vi "ArmMotorControl.vi"(8 "error in":errorcluster) -> ()   [LabVIEW 2014]
uses:
  Gantry/GantryGlobals.vi
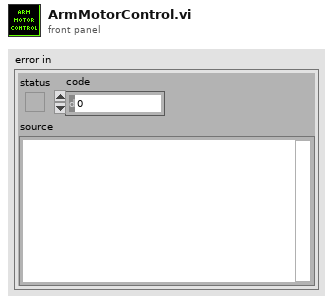
[diagram p1: front panel]
types:
  T1 = typedef "WPI_MotorControlDeviceRef.ctl" = cluster{"DeviceStatus":errorcluster, "Type":T2, "PWM":cluster{"Controller":T3, "PWM Channel":T4, "DeadBand":T5}, "CAN":cluster{"Device Number":u8, "Control Mode":T6, "Semaphore":T7, "Max Vout":dbl, "TalonSRX Control Mode":T8}, "Invert":bool, "TransformRef":T9, "InvTransformRef":T9}
  T2 = typedef "WPI_MotorControlType.ctl" = enum16{"PWM", "CAN", "CANTalonSRX"}
  T3 = typedef "FPGA_TypedefDigitalModule.ctl" = enum16{"Controller 1"}
  T4 = typedef "FPGA_DIOPWMChannel.ctl" = enum8{"PWM 0", "PWM 1", "PWM 2", "PWM 3", "PWM 4", "PWM 5", "PWM 6", "PWM 7", "PWM 8", "PWM 9", "PWM MXP 0", "PWM MXP 1", "PWM MXP 2", "PWM MXP 3", "PWM MXP 4", "PWM MXP 5", "PWM MXP 6", "PWM MXP 7", "PWM MXP 8", "PWM MXP 9", "Invalid"}
  T5 = typedef "WPI_PWMDeadband.ctl" = cluster{"Name":string, "maxPositivePwm":i32, "minPositivePwm":i32, "centerPwm":i32, "maxNegativePwm":i32, "minNegativePwm":i32, "angularRange":u16}
  T6 = typedef "WPI_CANJaguar_ControlMode.ctl" = enum8{"Percent VBus", "Current", "Speed", "Position", "Voltage"}
  T7 = typedef "Semaphore RefNum" = refnum<k1>
  T8 = typedef "WPI_CANTalonSRX_APIControlMode.ctl" = enum8{"Percent VBus", "Speed", "Position", "Slave", "Unchanged / Invalid"}
  T9 = typedef "WPI_PWMTransform_ConPane.ctl" = refnum<vi>
  T10 = typedef "WPI_CANTalonSRX_GlobalStatus.ctl" = cluster{"Applied Throttle":dbl, "Module Enabled":bool, "CAN Error":errorcluster, "Closed Loop Error":dbl, "Forward Limit Switch Closed":bool, "Reverse Limit Switch Closed":bool, "Sensor Position":dbl, "Sensor Velocity":dbl, "Current":dbl, "Sticky Fault - Over Temp":bool, "Sticky Fault - Under Voltage":bool, "Sticky Fault - Forward Limit":bool, "Sticky Fault - Reverse Limit":bool, "Sticky Fault - Forward Soft Limit":bool, "Sticky Fault - Reverse Soft Limit":bool, "Brake is Enabled":bool, "Encoder Position":dbl, "Encoder Velocity":dbl, "Encoder Index Count":dbl, "Encoder A Pin State":bool, "Encoder B Pin State":bool, "Encoder Index Pin State":bool, "Analog In":dbl, "Analog In Velocity":dbl, "Temperature (C)":dbl, "Battery Voltage":dbl}
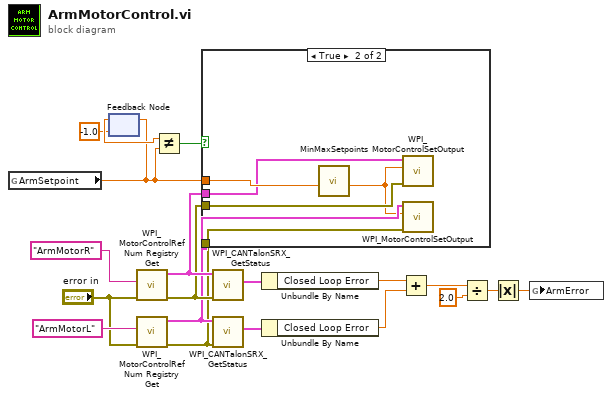
[diagram p0: block diagram]
diagram:
  n1 = global read "GantryGlobals.vi" "ArmSetpoint"() -> (w1:dbl)
  n2 = feedback-in #1(w1) -> ()
  n3 = feedback #1(-1.0 ("ArmSetpoint")) -> (w3:dbl)
  n4 = call <vilib>:"WPI_MotorControlRefNum Registry Get.vi"("error in (no error)"="error in", "refnum name"="ArmMotorR") -> ("error out"=w15:errorcluster, "MotorControlDevRef"=w16:T1)  [unwired: 8 in]
  n5 = call <vilib>:"WPI_MotorControlRefNum Registry Get.vi"("error in (no error)"="error in", "refnum name"="ArmMotorL") -> ("error out"=w13:errorcluster, "MotorControlDevRef"=w14:T1)  [unwired: 8 in]
  n6 = Not Equal?(x=w3, y=w1) -> (x != y?=w4:bool)
  n7 = case shown="True" w4 {
    tunnel: w1 -> [_ w25]
    tunnel: w16 -> [_ w24]
    tunnel: w15 -> [_ w23]
    tunnel: w14 -> [_ w22]
    tunnel: w13 -> [_ w21]
    frame False {
    }
    frame True {
      n8 = call "MinMaxSetpoints.vi"("ArmIn"=w25) -> ("ArmOut"=w20:dbl)  [unwired: 8 in, 2 out]
      n9 = call <vilib>:"WPI_MotorControlSetOutput.vi"("error in (no error)"=w23, "Output"=w20, "MotorControlDevRef"=w24) -> ()  [unwired: 6 in, 3 out]
      n10 = call <vilib>:"WPI_MotorControlSetOutput.vi"("error in (no error)"=w21, "Output"=w20, "MotorControlDevRef"=w22) -> ()  [unwired: 6 in, 3 out]
    }
  }
  n11 = call <vilib>:"WPI_CANTalonSRX_GetStatus.vi"("error in (no error)"=w15, "CAN Talon SRX Ref"=w16) -> ("Talon SRX Status"=w12:T10)  [unwired: 7 in, 2 out]
  n12 = call <vilib>:"WPI_CANTalonSRX_GetStatus.vi"("error in (no error)"=w13, "CAN Talon SRX Ref"=w14) -> ("Talon SRX Status"=w11:T10)  [unwired: 7 in, 2 out]
  n13 = Unbundle By Name(w12) -> ("Closed Loop Error"=w10:dbl)
  n14 = Unbundle By Name(w11) -> ("Closed Loop Error"=w9:dbl)
  n15 = Add(x=w10, y=w9) -> (x+y=w8:dbl)
  n16 = Divide(x=w8, y=2.0) -> (x/y=w6:dbl)
  n17 = Absolute Value(x=w6) -> (abs(x)=w5:dbl)
  n18 = global write "GantryGlobals.vi" "ArmError"(w5) -> ()
